vi "numeric_invalididentifiers.vi"(11 "x in":dbl) -> (3 "y out":dbl)   [LabVIEW 2020]
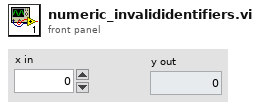
[diagram p1: front panel]
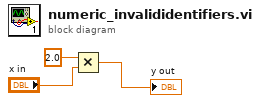
[diagram p0: block diagram]
diagram:
  n1 = Multiply(x=2.0, y="x in") -> (x*y=→"y out":dbl)
